vi "Read FPGA VI Reference.vi"(8 "error in (no error)":errorcluster, 11 "AODAcq in":refnum<class "AODAcq.lvclass">) -> (0 "error out":errorcluster, 2 "FPGA VI Reference":T1, 3 "AODAcq out":refnum<class "AODAcq.lvclass">)   [LabVIEW 2014, in "AODAcq.lvclass"]
uses:
  AODAcq.lvclass
  FPGA_Control/AODRef.ctl
  AODAcq.lvclass/AODAcq.ctl
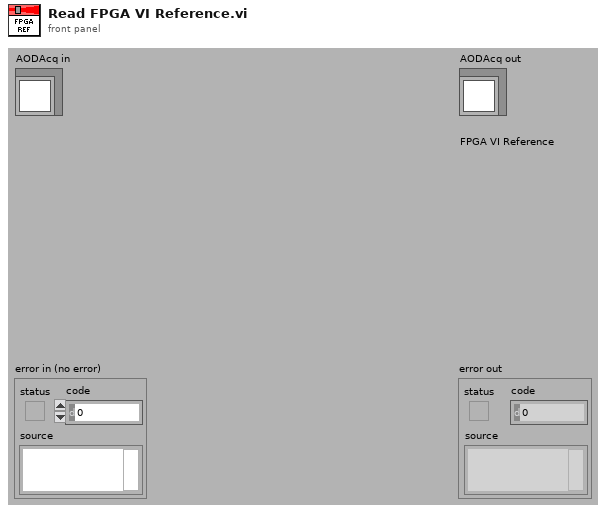
[diagram p1: front panel]
types:
  T1 = typedef "AODRef.ctl" = refnum<k20>
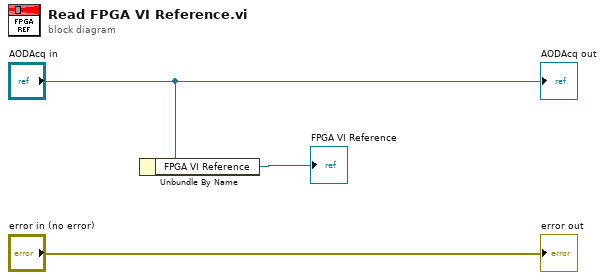
[diagram p0: block diagram]
diagram:
  n1 = Unbundle By Name("AODAcq in") -> ("FPGA VI Reference"=→"FPGA VI Reference":T1)
  "error out" <- "error in (no error)"
  "AODAcq out" <- "AODAcq in"
